vi "start.vi"(8 "error in (no error)":errorcluster, 11 "DL090211DAQScaffold in":refnum<class "DAQ_MG090622Camera.lvclass">) -> (0 "error out":errorcluster, 3 "DL090211DAQScaffold out":refnum<class "DAQ_MG090622Camera.lvclass">)   [LabVIEW 2010, in "DAQ_MG090622Camera.lvclass"]
uses:
  DAQ_MG090622Camera.lvclass
  DAQ_DL090211Scaffold/DAQ_DL090211Scaffold/DAQ_DL090211Scaffold.lvclass
  DAQ_MG090622Camera.lvclass/DAQ_MG090622Camera.ctl
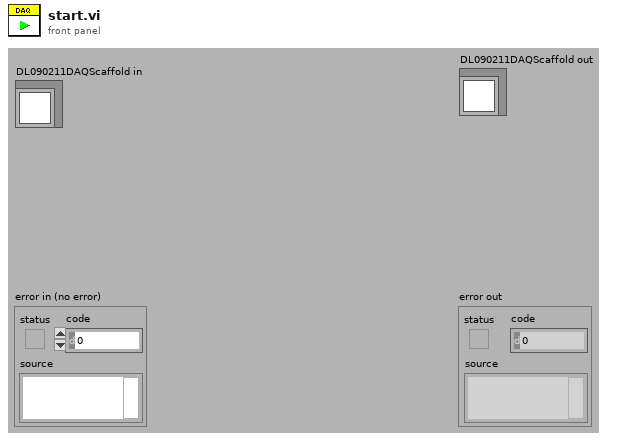
[diagram p1: front panel]
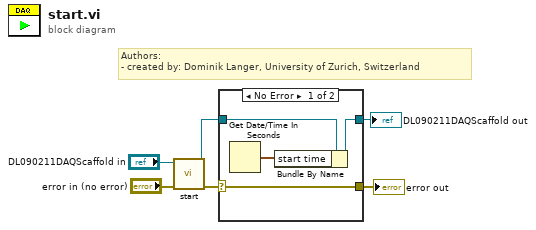
[diagram p0: block diagram]
diagram:
  # "Authors: \n- created by: Dominik Langer, University of Zurich, Switzerland"
  n1 = call-parent "start.vi"("error in (no error)"="error in (no error)", "DL090211DAQScaffold in"="DL090211DAQScaffold in") -> ("error out"=w4:errorcluster, "DL090211DAQScaffold out"=w3:refnum<class "DAQ_MG090622Camera.lvclass">)  [unwired: 8 in]
  n2 = case shown="No Error" w4 {
    selector: w4 -> [w10 w12]
    tunnel: w3 -> [w8 w11]
    tunnel: [w10 w12] -> w1
    tunnel: [w7 w11] -> w2
    frame No Error {
      n3 = Get Date/Time In Seconds() -> (seconds since 1Jan1904=w9:timestamp)
      n4 = Bundle By Name(cluster=w8, "start time"=w9) -> (w7:refnum<class "DAQ_MG090622Camera.lvclass">)
    }
    frame Error {
    }
  }
  "error out" <- w1
  "DL090211DAQScaffold out" <- w2
